vi "Get_Error_Code.vi"(0 "Logger_Data":T1) -> (4 "Error_Code":u32)   [LabVIEW 2023]
doc: "Used to get the Error code from the generated data and limits."
uses:
  Controls/Logger_Data.ctl
  Controls/Generated_data.ctl
  Controls/Current_Limit.ctl
  Controls/Temperature_Limit.ctl
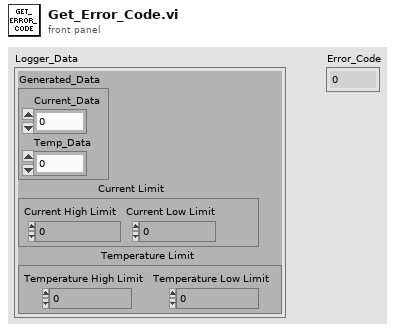
[diagram p1: front panel]
types:
  T1 = typedef "Logger_Data.ctl" = cluster{"Generated_Data":T2, "Current_Limit":T3, "Temperature_Limit":T4}
  T2 = typedef "Generated_data.ctl" = cluster{"Current_Data":dbl, "Temp_Data":dbl}
  T3 = typedef "Current_Limit.ctl" = cluster{"Current_High_Limit":dbl, "Current_Low_Limit":dbl}
  T4 = typedef "Temperature_Limit.ctl" = cluster{"Temperature_High_Limit":dbl, "Temperature_Low_Limit":dbl}
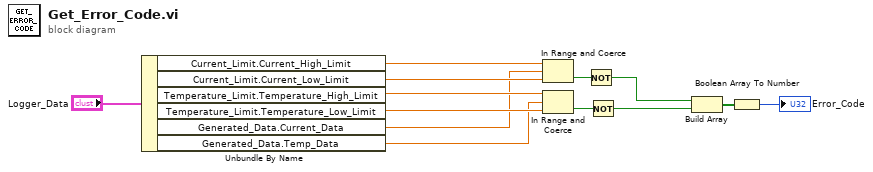
[diagram p0: block diagram]
diagram:
  n1 = Unbundle By Name("Logger_Data") -> ("Current_Limit.Current_High_Limit"=w4:dbl, "Current_Limit.Current_Low_Limit"=w2:dbl, "Temperature_Limit.Temperature_High_Limit"=w8:dbl, "Temperature_Limit.Temperature_Low_Limit"=w9:dbl, "Generated_Data.Current_Data"=w1:dbl, "Generated_Data.Temp_Data"=w7:dbl)
  n2 = In Range and Coerce(upper limit=w4, x=w1, lower limit=w2) -> (In Range?=w10:bool)  [unwired: 1 out]
  n3 = In Range and Coerce(upper limit=w8, x=w7, lower limit=w9) -> (In Range?=w11:bool)  [unwired: 1 out]
  n4 = Not(x=w10) -> (.not. x?=w6:bool)
  n5 = Not(x=w11) -> (.not. x?=w5:bool)
  n6 = Build Array(w6, w5) -> (w12:bool[])
  n7 = Boolean Array To Number(Boolean array=w12) -> (number=→"Error_Code":u32)
